vi "String.vi"() -> ()   [LabVIEW 2020]
panel:
  out "decimal integer string 2":string
  out "F-format string":string
  out "decimal integer string":string
  in  "Boolean":bool
  in  "Thermometer":dbl(slide) scale=0.0..100.0
  in  "Tank":u16(slide) scale=0.0..10.0
  out "Output":string
  in  "Enter":bool
  in  "Ingrese su Apellido":string
  in  "Ingrese su Nombre":string
  out "all upper case string":string
  out "all lower case string":string
  out "substring":string
  out "concatenated string":string
  out "length":i32
  out "Dato B":string
  in  "Dato A":string
  # "String"
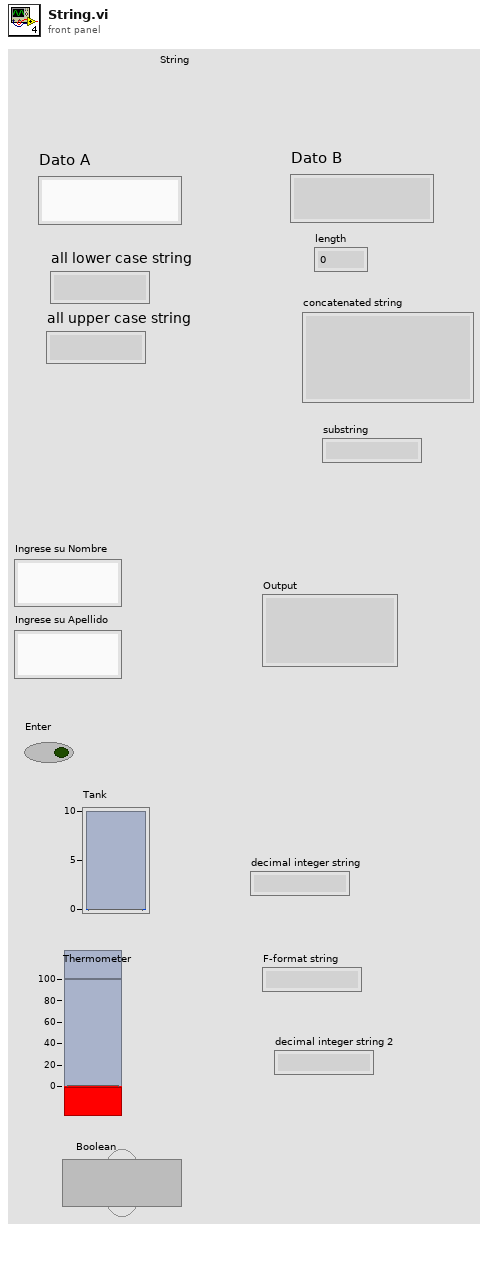
[diagram p1: front panel]
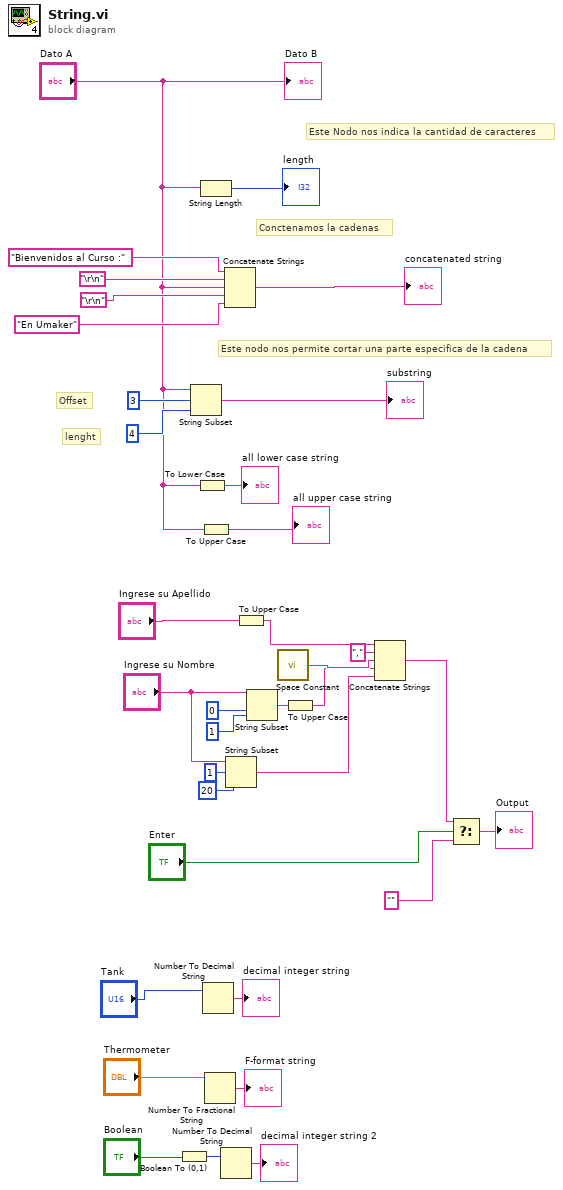
[diagram p0: block diagram]
diagram:
  # "Este nodo nos permite cortar una parte especifica de la cadena"
  # "Conctenamos la cadenas"
  # "lenght"
  # "Offset"
  # "Este Nodo nos indica la cantidad de caracteres"
  n1 = Boolean To (0,1)(Boolean="Boolean") -> (0, 1=w4:i16)
  n2 = String Subset(string="Dato A", offset (0)=3, length (rest)=4 ("length (rest)")) -> (substring=→"substring":string)
  n3 = To Lower Case(string="Dato A") -> (all lower case string=→"all lower case string":string)
  n4 = String Length(string="Dato A") -> (length=→"length":i32)
  n5 = To Upper Case(1:"Dato A") -> (0:→"all upper case string":string)
  n6 = Number To Decimal String(number="Tank") -> (decimal integer string=→"decimal integer string":string)  [unwired: 1 in]
  n7 = Number To Fractional String(number="Thermometer") -> (F-format string=→"F-format string":string)  [unwired: 3 in]
  n8 = Number To Decimal String(number=w4) -> (decimal integer string=→"decimal integer string 2":string)  [unwired: 1 in]
  n9 = Concatenate Strings("Bienvenidos al Curso :", "\r\n", "Dato A", "\r\n", "En Umaker") -> (→"concatenated string":string)
  n10 = String Subset(string="Ingrese su Nombre", offset (0)=1, length (rest)=20 ("length (rest)")) -> (substring=w12:string)
  n11 = To Upper Case(1:"Ingrese su Apellido") -> (0:w16:string)
  n12 = String Subset(string="Ingrese su Nombre", offset (0)=0, length (rest)=1 ("length (rest)")) -> (substring=w17:string)
  n13 = call <vilib>:"Space Constant.vi"() -> ("String"=w14:string)
  n14 = To Upper Case(1:w17) -> (0:w13:string)
  n15 = Concatenate Strings(w16, "," ("string"), w14, w13, w12) -> (w10:string)
  n16 = Select(t=w10, s="Enter", f="") -> (s? t:f=→"Output":string)
  "Dato B" <- "Dato A"
